vi "RCM Open Running VI MHLC.vi"(8 "error in (no error)":errorcluster, 10 "Data":variant, 11 "Message Log in":refnum<class "Message Log.lvclass">) -> (0 "error out":errorcluster, 3 "Message Log out":refnum<class "Message Log.lvclass">)   [LabVIEW 2017, in "Message Log.lvclass"]
doc: "Open the front panel of the selected running Worker's Main VI"
uses:
  Message Log.lvclass
  Message Log.lvclass/Message Log.ctl
  rql_RCM Open Running VI.ctl
  Listbox Selection.ctl
  <vilib>/Utility/miscctls.llb/LVRowAndColumnTypeDef.ctl
  rsp_Open Running VI.ctl
  Common VIs/Message Log ID.ctl
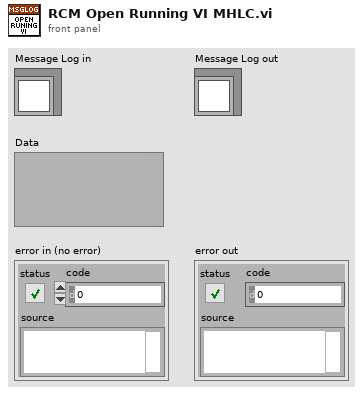
[diagram p1: front panel]
types:
  T1 = typedef "Message Log.lvclass/rql_RCM Open Running VI.ctl" = cluster{"Listbox Selection":T2}
  T2 = typedef "Message Log.lvclass/Listbox Selection.ctl" = cluster{"Cell Position":T3, "Row":string[]}
  T3 = typedef "LVRowAndColumnTypeDef.ctl" = cluster{"Row":i32, "Column":i32}
  T4 = typedef "Message Log.lvclass/rsp_Open Running VI.ctl" = cluster{"Message Log ID":T5, "Worker ID":string}
  T5 = typedef "Message Log ID.ctl" = cluster{"Head Worker ID":string, "IP Address":string}
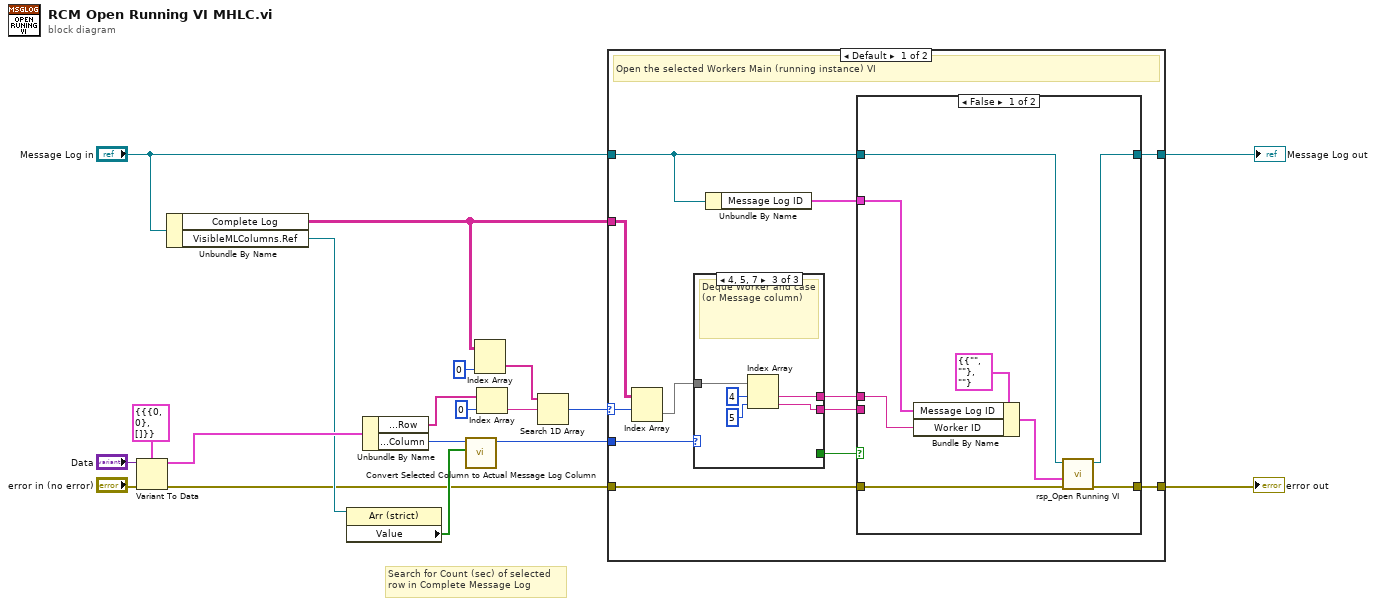
[diagram p0: block diagram]
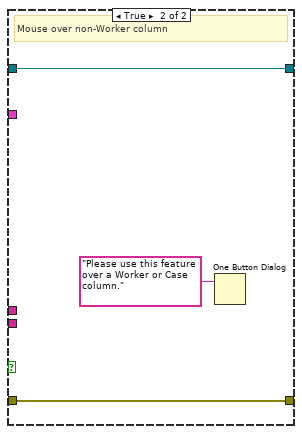
[diagram p2: hidden frame]
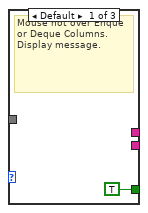
[diagram p3: hidden frame]
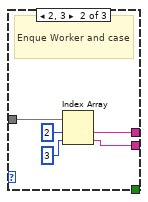
[diagram p4: hidden frame]
diagram:
  # "Search for Count (sec) of selected\nrow in Complete Message Log"
  n1 = Variant To Data(error in="error in (no error)", type=T1 {"Listbox Selection"={"Cell Position"={"Row"=0, "Column"=0}, "Row"=[]}} ("Data"), Variant="Data") -> (data=w10:T1, error out=w7:errorcluster)
  n2 = Unbundle By Name("Message Log in") -> ("Complete Log"=w4:string[][], "VisibleMLColumns.Ref"=w9:refnum<vi>)
  n3 = property class="Arr (strict)"(reference=w9) -> ("Value"=w8:bool[])  [unwired: 1 in, 2 out]
  n4 = Unbundle By Name(w10) -> ("Listbox Selection.Row"=w16:string[], "Listbox Selection.Cell Position.Column"=w11:i32)
  n5 = call "Convert Selected Column to Actual Message Log Column.vi"("Visible ML Columns"=w8, "Selected Column"=w11) -> ("Actual Column"=w6:i32)  [unwired: 9 in]
  n6 = Index Array(array=w4, index (col)=0 ("disabled index (col)")) -> (element=w12:string[])  [unwired: 1 in]
  n7 = Index Array(array=w16, index=0) -> (element=w13:string)
  n8 = Search 1D Array(1D array=w12, element=w13) -> (index of element=w5:i32)  [unwired: 1 in]
  n9 = case shown="Default" w5 {
    selector: w5 -> [w28 _]
    tunnel: [w26 w55] -> w1
    tunnel: w7 -> [w25 w55]
    tunnel: w4 -> [w31 _]
    tunnel: w6 -> [w30 _]
    tunnel: [w23 w54] -> w2
    tunnel: "Message Log in" -> [w24 w54]
    frame Default {
      # "Open the selected Workers Main (running instance) VI"
      n10 = Index Array(array=w31, index (row)=w28) -> (element=w29:string[])  [unwired: 1 in]
      n11 = case shown="4, 5, 7" w30 {
        tunnel: w29 -> [_ w47 w52]
        tunnel: [_ w46 w51] -> w21
        tunnel: [TRUE _ _] -> w27
        tunnel: [_ w44 w50] -> w20
        frame Default {
          # "Mouse not over Enque or Deque Columns.\nDisplay message."
        }
        frame 2, 3 {
          # "Enque Worker and case"
          n12 = Index Array(array=w47, index #1=2 ("index"), index #2=3 ("index")) -> (element #1=w46:string, element #2=w44:string)
        }
        frame 4, 5, 7 {
          # "Deque Worker and case (or Message column)"
          n13 = Index Array(array=w52, index #1=4 ("index"), index #2=5 ("index")) -> (element #1=w51:string, element #2=w50:string)
        }
      }
      n14 = Unbundle By Name(w24) -> ("Message Log ID"=w22:T5)
      n15 = case shown="False" w27 {
        tunnel: [w34 w41] -> w26
        tunnel: w25 -> [w35 w41]
        tunnel: w24 -> [w37 w40]
        tunnel: [w36 w40] -> w23
        tunnel: w22 -> [w33 _]
        tunnel: w21 -> [w32 _]
        tunnel: w20 -> [_ _]
        frame False {
          n16 = Bundle By Name(cluster=T4 {"Message Log ID"={"Head Worker ID"="", "IP Address"=""}, "Worker ID"=""} ("Data in"), "Message Log ID"=w33, "Worker ID"=w32) -> (w38:T4)
          n17 = call "rsp_Open Running VI.vi"("error in"=w35, "Data in"=w38, "Message Log in"=w37) -> ("error out"=w34:errorcluster, "dup Message Log out"=w36:refnum<class "Message Log.lvclass">)  [unwired: 7 in]
        }
        frame True {
          # "Mouse over non-Worker column"
          n18 = One Button Dialog(message="Please use this feature over a Worker or Case column.") -> ()  [unwired: 1 in, 1 out]
        }
      }
    }
    frame -1 {
      # "Can't find Row in complete message log\nPossible that this row doesn't exist in the Complete message log any longer. Do nothing"
    }
  }
  "Message Log out" <- w2
  "error out" <- w1
